vi "WaitForSegs.vi"(0 "Acqiris ID":u32, 2 "lines per plane":i32, 3 "error in":errorcluster, 4 "Timeout":i32=1000) -> (5 "dup Instrument ID":u32, 6 "status":bool, 7 "error out":errorcluster)   [LabVIEW 2022 SP3]
uses:
  <vilib>/Platform/TimedLoop/XDataNode/timing_clust.ctl
  <vilib>/Platform/TimedLoop/XDataNode/nitl_modes.ctl
  <vilib>/Platform/TimedLoop/XDataNode/wakeup.ctl
  <vilib>/Platform/TimedLoop/XDataNode/XDataNode.xnode
  <instrlib>/Acqiris Dx/Acqiris Dx.lvlib
  <vilib>/Platform/TimedLoop/XDataNode/XDNodeRunTimeDep.lvlib
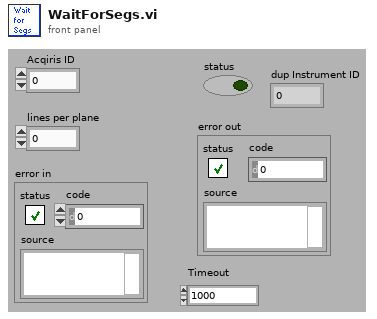
[diagram p1: front panel]
types:
  T1 = typedef "XDNodeRunTimeDep.lvlib/timing_clust.ctl" = cluster{"Expected End [f-1]":u64, "Actual End [f-1]":u64, "Finished Late? [f-1]":bool, "Expected End [i-1]":u64, "Actual End [i-1]":u64, "Finished Late? [i-1]":bool, "Expected Start [i]":u64, "Actual Start [i]":u64, "Expected Start [f]":u64, "Actual Start [f]":u64, "Source Name":string, "Structure Name":string, "Period":i64, "Deadline":i64, "Offset":i64, "Start":i64, "Priority":i32, "Timeout":i32, "Mode":T2, "Wakeup Reason":T3, "Error":errorcluster, "Source Type":string, "Secondary Source Type":string, "Global End Time":u64, "Global Start Time":u64, "Frame Duration":u64, "Iteration Duration":u64, "Assigned CPU":i32, "I/O Scan Engine Mode":u32}
  T2 = typedef "XDNodeRunTimeDep.lvlib/nitl_modes.ctl" = enum32{"No Change", "Process missed periods, maintain original phase", "Discard missed periods, maintain original phase", "Process missed periods, ignore original phase", "Discard missed periods, ignore original phase"}
  T3 = typedef "XDNodeRunTimeDep.lvlib/wakeup.ctl" = enum32{"Normal", "Aborted", "Asynchronous wakeup", "Timing source error", "Timed loop error", "Timeout"}
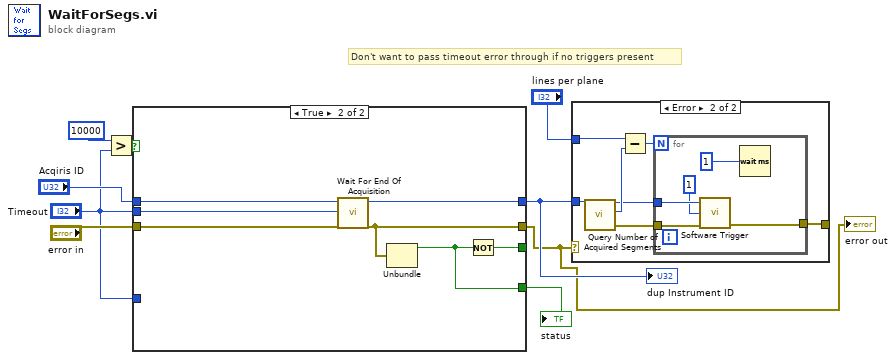
[diagram p0: block diagram]
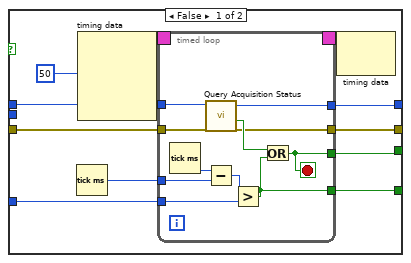
[diagram p2: hidden frame]
diagram:
  # "Don't want to pass timeout error through if no triggers present"
  n1 = Greater?(x=10000, y="Timeout") -> (0:w5:bool)
  n2 = case shown="True" w5 {
    tunnel: "Acqiris ID" -> [w20 w44]
    tunnel: "Timeout" -> [_ w43]
    tunnel: [w10 w38] -> _
    tunnel: "error in" -> [w18 w42]
    tunnel: [w19 w41] -> w2
    tunnel: [w15 w40] -> w1
    tunnel: "Timeout" -> [w16 _]
    tunnel: [w11 w39] -> w3
    frame False {
      n3 = Tick Count (ms)() -> (millisecond timer value=w17:u32)
      n4 = node-c288(i64 50 ("Period")) -> (w14:T1)  [unwired: 3 in]
      n5 = timed-loop {
        tunnel: w20 -> [w31]
        tunnel: [w30] -> w19
        tunnel: w18 -> [w29]
        tunnel: [w22] -> w10
        tunnel: w17 -> [w26]
        tunnel: w16 -> [w24]
        tunnel: [w23] -> w15
        timing: w14 -> [_]
        timing-out: [_] -> w13
        tunnel: [w21] -> w11
        stop <- w22 stop-if-true
        n6 = Tick Count (ms)() -> (millisecond timer value=w27:u32)
        n7 = call <instrlib>:"Query Acquisition Status.vi"("error in (no error)"=w29, "Instrument ID"=w31) -> ("error out"=w23:errorcluster, "Done?"=w28:bool, "dup Instrument ID"=w30:u32)  [unwired: 2 in, 1 out]
        n8 = Subtract(x=w27, y=w26) -> (x-y=w25:u32)
        n9 = Greater?(x=w25, y=w24) -> (0:w21:bool)
        n10 = Or(x=w28, y=w21) -> (x .or. y?=w22:bool)
      }
      n11 = node-c288(w13) -> ()  [unwired: 1 out]
    }
    frame True {
      n12 = call <instrlib>:"Wait For End Of Acquisition.vi"("error in (no error)"=w42, "Timeout"=w43, "Instrument ID"=w44) -> ("error out"=w40:errorcluster, "dup Instrument ID"=w41:u32)  [unwired: 3 out]
      n13 = Unbundle(w40) -> ("status"=w39:bool)  [unwired: 2 out]
      n14 = Not(x=w39) -> (.not. x?=w38:bool)
    }
  }
  "error out" <- w1
  "status" <- w3
  "dup Instrument ID" <- w2
  n15 = case shown="Error" w1 {
    tunnel: w2 -> [_ w51]
    tunnel: "lines per plane" -> [_ w50]
    tunnel: [_ w45] -> _
    frame No Error {
    }
    frame Error {
      n16 = call <instrlib>:"Query Number of Acquired Segments.vi"("Instrument ID"=w51) -> ("error out"=w46:errorcluster, "Number of Segments"=w49:i32, "dup Instrument ID"=w47:u32)  [unwired: 1 in, 3 out]
      n17 = Subtract(x=w50, y=w49) -> (x-y=w48:i32)
      n18 = for {
        N: w48 -> [_]
        tunnel: w46 -> [w56]
        tunnel: w47 -> [w55]
        tunnel: [w53] -> w45
        n19 = call <instrlib>:"Software Trigger.vi"("error in (no error)"=w56, "Type"=1, "Instrument ID"=w55) -> ("error out"=w53:errorcluster)  [unwired: 1 out]
        n20 = Wait (ms)(milliseconds to wait=1) -> ()  [unwired: 1 out]
      }
    }
  }
